vi "AlliGator Paths.vi"(6 "Get(F)/Set":bool, 8 "error in (no error)":errorcluster, 11 "AlliGator.vi Path":path) -> (0 "error out":errorcluster, 1 "Data Folder":path, 2 "Python Plugins Folder":path, 3 "GUI Folder":path, 5 "AlliGator Folder":path)   [LabVIEW 2021, in "AlliGator GUI.lvlib"]
doc: "Stores folder paths used throughout AlliGator."
uses:
  AlliGator GUI.lvlib
panel:
  # "see the AlliGator License on the block diagram (Ctrl+E or Window:Show Block Diagram)"
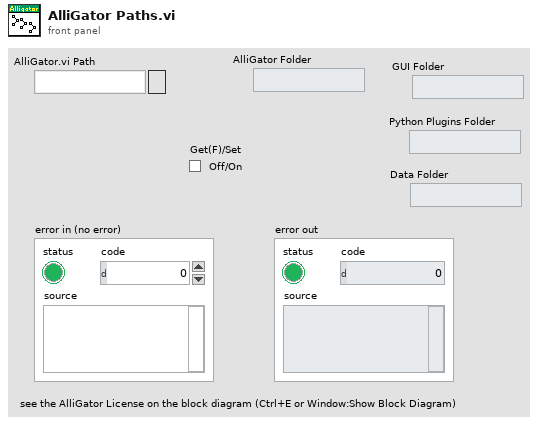
[diagram p1: front panel]
types:
  T1 = enum32{"invalid app kind", "Development System", "Run Time System", "Student Edition", "Embedded LabVIEW", "Evaluation", "Custom"}
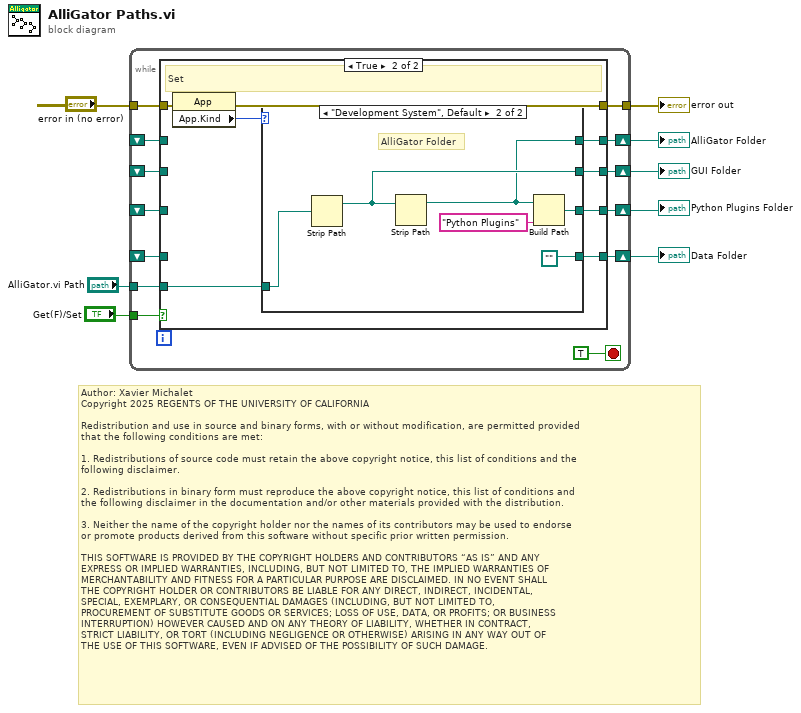
[diagram p0: block diagram]
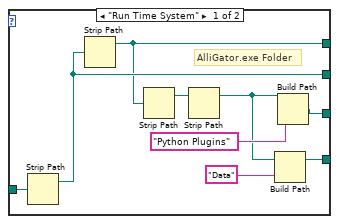
[diagram p3: hidden frame]
diagram:
  # "Author: Xavier Michalet\nCopyright 2025 REGENTS OF THE UNIVERSITY OF CALIFORNIA\n\nRedistribution and use in source and binary forms, with or without modification, are permitted provided\nthat the following conditions are met:\n\n1. Redistributions of source code must retain the above copyright notice, this list of conditions and the\nfollowing disclaimer.\n\n2. Redistributions in binary form must reproduce the above copyright notice, this list of conditions and\nthe following disclaimer in the documentation and/or other materials provided with the distribution.\n\n3. Neither the name of the copyright holder nor the names of its contributors may be used to endorse \nor promote products derived from this software without specific prior written permission.\n\nTHIS SOFTWARE IS PROVIDED BY THE COPYRIGHT HOLDERS AND CONTRIBUTORS “AS IS” AND ANY \nEXPRESS OR IMPLIED WARRANTIES, INCLUDING, BUT NOT LIMITED TO, THE IMPLIED WARRANTIES OF\nMERCHANTABILITY AND FITNESS FOR A PARTICULAR PURPOSE ARE DISCLAIMED. IN NO EVENT SHALL\nTHE COPYRIGHT HOLDER OR CONTRIBUTORS BE LIABLE FOR ANY DIRECT, INDIRECT, INCIDENTAL, \nSPECIAL, EXEMPLARY, OR CONSEQUENTIAL DAMAGES (INCLUDING, BUT NOT LIMITED TO, \nPROCUREMENT OF SUBSTITUTE GOODS OR SERVICES; LOSS OF USE, DATA, OR PROFITS; OR BUSINESS\nINTERRUPTION) HOWEVER CAUSED AND ON ANY THEORY OF LIABILITY, WHETHER IN CONTRACT, \nSTRICT LIABILITY, OR TORT (INCLUDING NEGLIGENCE OR OTHERWISE) ARISING IN ANY WAY OUT OF\nTHE USE OF THIS SOFTWARE, EVEN IF ADVISED OF THE POSSIBILITY OF SUCH DAMAGE."
  n1 = while {
    shift-right: [w20] -> w7
    shift-left: _ -> [w10]
    tunnel: "AlliGator.vi Path" -> [w14]
    tunnel: "error in (no error)" -> [w19]
    tunnel: [w18] -> w5
    tunnel: "Get(F)/Set" -> [w13]
    shift-right: [w16] -> w3
    shift-left: _ -> [w12]
    shift-right: [w21] -> w8
    shift-left: _ -> [w11]
    shift-right: [w17] -> w4
    shift-left: _ -> [w9]
    stop <- TRUE stop-if-true
    n2 = case shown="True" w13 {
      tunnel: [w24 w33] -> w21
      tunnel: [w23 w32] -> w20
      tunnel: w19 -> [w25 w31]
      tunnel: [w25 w30] -> w18
      tunnel: [w22 w29] -> w17
      tunnel: [w26 w28] -> w16
      tunnel: w14 -> [_ w27]
      tunnel: w12 -> [w26 _]
      tunnel: w11 -> [w24 _]
      tunnel: w10 -> [w23 _]
      tunnel: w9 -> [w22 _]
      frame False {
        # "Get"
      }
      frame True {
        # "Set"
        n3 = property class="App"(error in=w31) -> (error out=w30:errorcluster, "App.Kind"=w34:T1)  [unwired: 1 in, 1 out]
        n4 = case shown="\"Development System\", Default" w34 {
          tunnel: [w38 w49] -> w33
          tunnel: [w42 w47] -> w32
          tunnel: [w40 path ""] -> w29
          tunnel: [w37 w45] -> w28
          tunnel: w27 -> [w39 w44]
          frame "Run Time System" {
            # "AlliGator.exe Folder"
            n5 = Strip Path(path=w39) -> (stripped path=w38:path)  [unwired: 1 out]
            n6 = Strip Path(path=w38) -> (stripped path=w37:path)  [unwired: 1 out]
            n7 = Strip Path(path=w37) -> (stripped path=w36:path)  [unwired: 1 out]
            n8 = Strip Path(path=w36) -> (stripped path=w35:path)  [unwired: 1 out]
            n9 = Build Path(base path=w35, name or relative path="Data" ("name")) -> (appended path=w40:path)
            n10 = Build Path(base path=w35, name or relative path="Python Plugins" ("name")) -> (appended path=w42:path)
          }
          frame "Development System", Default {
            # "AlliGator Folder"
            n11 = Strip Path(path=w44) -> (stripped path=w49:path)  [unwired: 1 out]
            n12 = Strip Path(path=w49) -> (stripped path=w45:path)  [unwired: 1 out]
            n13 = Build Path(base path=w45, name or relative path="Python Plugins" ("name")) -> (appended path=w47:path)
          }
        }
      }
    }
  }
  "Python Plugins Folder" <- w7
  "GUI Folder" <- w8
  "error out" <- w5
  "Data Folder" <- w4
  "AlliGator Folder" <- w3
